vi "Time-Delayed Send Message Core.vi"(4 "Caller Info":cluster{"Clone Type":string, "Clone ID":string}, 6 "Message Priority (Normal)":T1=enum."Normal", 7 "How Many Copies (0 = infinite repeat)":u32, 8 "Time To Wait":i32=1000, 9 "Delivery Notifier":refnum<notifier>, 10 "Message":refnum<class "Message.lvclass">, 11 "Message Enqueuer":refnum<class "Message Enqueuer.lvclass">) -> ()   [LabVIEW 2017, in "AF_Messages-PPL.lvlib"]
doc: "This VI forms the core processing loop for the time-delayed messages. This VI may be called directly if the desired behavior is for the caller to wait until the messages have been sent before continuing, but the usual usage of this VI is to call <b>Time-Delayed Send Message.vi</b> which will launch an asynch clone of this VI so that the caller can proceed with other work instead of waiting for the time out. \n\nSee Context Help for <b>Time-Delayed Send Message.vi</b> for further details."
uses:
  AF_Messages-PPL.lvlib
  Actor Framework.lvlibp/Message Enqueuer/Message Enqueuer.lvclass
  Actor Framework.lvlibp/Message/Message.lvclass
  <vilib>/ActorFramework/Time-Delayed Send Message/Time-Delay Override Options.ctl
  Actor Framework.lvlibp/Message Enqueuer/Message Priority.ctl
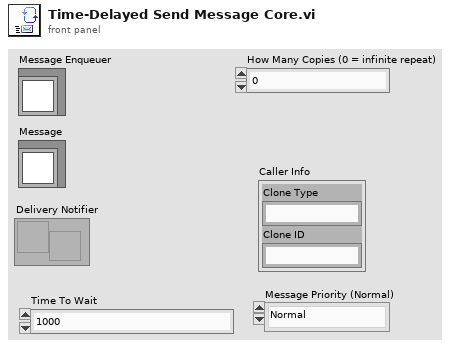
[diagram p1: front panel]
types:
  T1 = typedef "Actor Framework.lvlibp/Message Enqueuer.lvclass/Message Priority.ctl" = enum16{"Low", "Normal", "High"}
  T2 = typedef "Time-Delay Override Options.ctl" = enum16{"Send next copy now", "Skip next scheduled copy", "Send next copy now and stop all further copies", "Stop all further copies"}
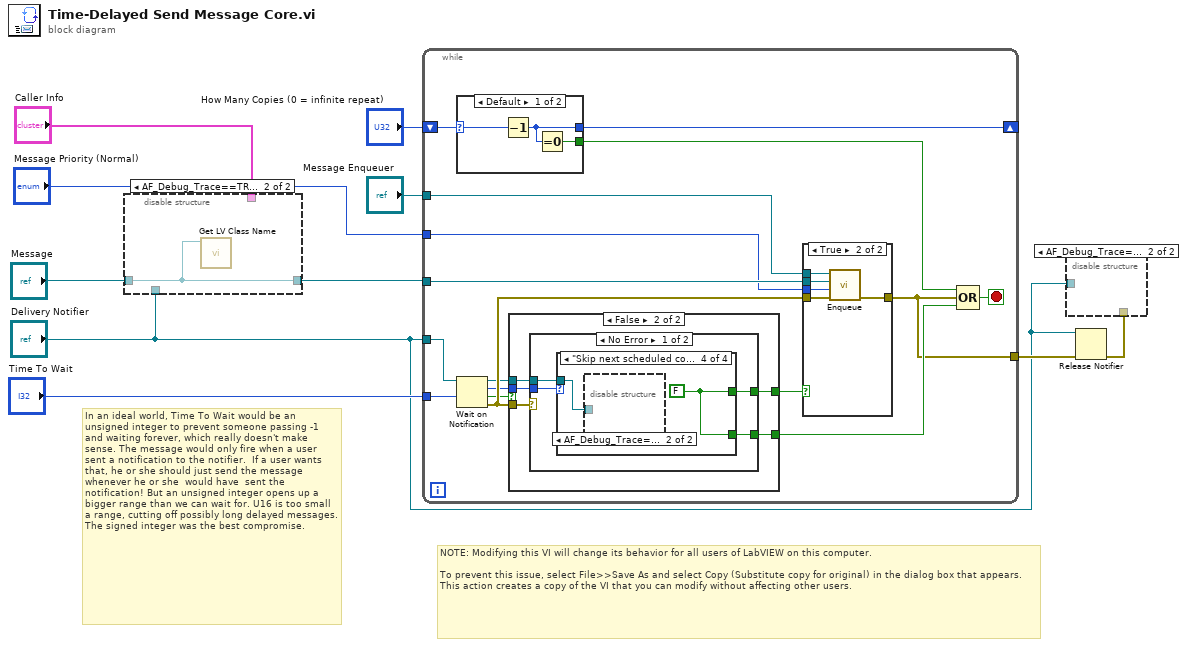
[diagram p0: block diagram]
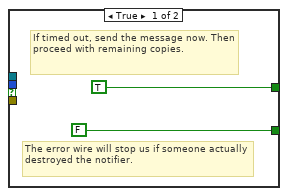
[diagram p4: hidden frame]
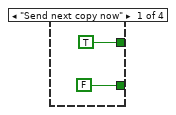
[diagram p5: hidden frame]
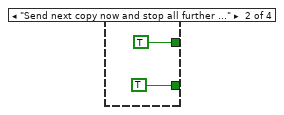
[diagram p6: hidden frame]
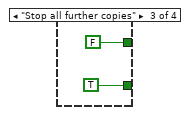
[diagram p7: hidden frame]
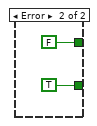
[diagram p9: hidden frame]
diagram:
  # "NOTE: Modifying this VI will change its behavior for all users of LabVIEW on this computer.\n\nTo prevent this issue, select File>>Save As and select Copy (Substitute copy for original) in the dialog box that appears. This action creates a copy of the VI that you can modify without affecting other users."
  # "In an ideal world, Time To Wait would be an unsigned integer to prevent someone passing -1 and waiting forever, which really doesn't make sense. The message would only fire when a user sent a notification to the notifier.  If a user wants that, he or she should just send the message whenever he or she  would have  sent the notification! But an unsigned integer opens up a bigger range than we can wait for. U16 is too small a range, cutting off possibly long delayed messages. The signed integer was the best compromise."
  n1 = disable-structure shown="AF_Debug_Trace==TRUE" {
    disable-tunnel: "Message" -> [w11 w13]
    disable-tunnel: [w11 w13] -> w4
    disable-tunnel: "Delivery Notifier" -> [_ w12]
    disable-tunnel: "Caller Info" -> [_ _]
    frame condition #0 (active) {
    }
    frame condition #1 {
      n2 = call <vilib>:"Get LV Class Name.vi"("object"=w13) -> ()  [unwired: 9 in, 2 out]
    }
  }
  n3 = while {
    shift-right: [w27] -> _
    shift-left: "How Many Copies (0 = infinite repeat)" -> [w28]
    tunnel: "Delivery Notifier" -> [w26]
    tunnel: "Message Enqueuer" -> [w25]
    tunnel: w4 -> [w24]
    tunnel: "Time To Wait" -> [w18]
    tunnel: [w16] -> w7
    tunnel: "Message Priority (Normal)" -> [w15]
    stop <- w23 stop-if-true
    n4 = case shown="Default" w28 {
      selector: w28 -> [w59 w60]
      tunnel: [w58 w60] -> w27
      tunnel: [w57 _] -> w22
      frame Default {
        n5 = Decrement(x=w59) -> (x-1=w58:u32)
        n6 = Equal To 0?(x=w58) -> (x = 0?=w57:bool)
      }
      frame 0 {
      }
    }
    n7 = Wait on Notification(notifier=w26, timeout in ms (-1)=w18) -> (notifier out=w14:refnum<notifier>, notification=w19:T2, timed out?=w21:bool, error out=w29:errorcluster)  [unwired: 2 in]
    n8 = case shown="False" w21 {
      tunnel: [TRUE w35] -> w20
      tunnel: w19 -> [_ w34]
      tunnel: w29 -> [_ w36]
      tunnel: [FALSE w33] -> w17
      tunnel: w14 -> [_ w32]
      frame True {
        # "The error wire will stop us if someone actually destroyed the notifier."
        # "If timed out, send the message now. Then proceed with remaining copies."
      }
      frame False {
        n9 = case shown="No Error" w36 {
          tunnel: [w39 FALSE] -> w35
          tunnel: w34 -> [w40 _]
          tunnel: [w38 TRUE] -> w33
          tunnel: w32 -> [w37 _]
          frame No Error {
            n10 = case shown="\"Skip next scheduled copy\"" w40 {
              tunnel: [TRUE TRUE FALSE w48] -> w39
              tunnel: [FALSE TRUE TRUE w48] -> w38
              tunnel: w37 -> [_ _ _ w47]
              frame "Send next copy now" {
              }
              frame "Send next copy now and stop all further copies" {
              }
              frame "Stop all further copies" {
              }
              frame "Skip next scheduled copy" {
                w48 = FALSE
                n11 = disable-structure shown="AF_Debug_Trace==TRUE" {
                  disable-tunnel: w47 -> [_ _]
                  frame condition #0 (active) {
                  }
                  frame condition #1 {
                  }
                }
              }
            }
          }
          frame Error {
          }
        }
      }
    }
    n12 = case shown="True" w20 {
      tunnel: w25 -> [_ w56]
      tunnel: w24 -> [_ w55]
      tunnel: w29 -> [w51 w54]
      tunnel: [w51 w53] -> w16
      tunnel: w15 -> [_ w52]
      frame False {
      }
      frame True {
        n13 = call "Enqueue.vi"("error in (no error)"=w54, "Message Priority (Normal)"=w52, "Message"=w55, "Message Enqueuer in"=w56) -> ("error out"=w53:errorcluster)  [unwired: 6 in, 1 out]
      }
    }
    n14 = Compound Arithmetic op=OR(w22, w16, w17) -> (w23:bool)
  }
  n15 = Release Notifier(notifier="Delivery Notifier", error in (no error)=w7) -> (error out=w1:errorcluster)  [unwired: 1 in, 2 out]
  n16 = disable-structure shown="AF_Debug_Trace==TRUE" {
    disable-tunnel: "Delivery Notifier" -> [_ _]
    disable-tunnel: w1 -> [_ _]
    frame condition #0 (active) {
    }
    frame condition #1 {
    }
  }
